vi "Read_Instr.vi"(8 "error in (no error)":errorcluster caption="entrée d'erreur (pas d'erreur)", 11 "Class Instrument Process en entrée":refnum<class "Class Instrument Process.lvclass">) -> (0 "error out":errorcluster caption="sortie d'erreur", 3 "Class Instrument Process en sortie":refnum<class "Class Instrument Process.lvclass">)   [LabVIEW 2020, in "Library Instrument & Equipement.lvlib" / "Library Instruments.lvlib" / "Class Instrument Process.lvclass"]
uses:
  Class Instrument Process.lvclass
  Class Instrument Process.lvclass/Class Instrument Process.ctl
  Instrument (Default)/Class Instrument (Default).lvclass
  Process/Process (Default)/Process (Default).lvclass
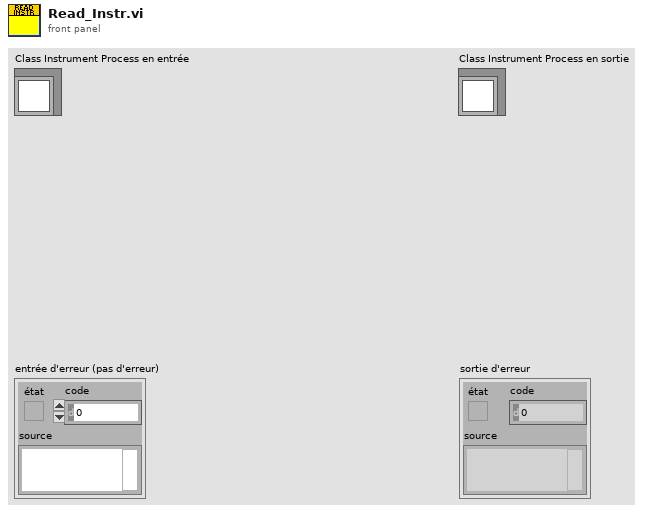
[diagram p1: front panel]
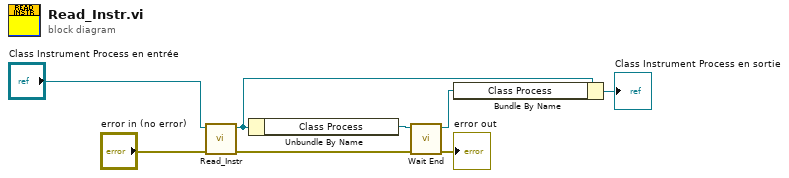
[diagram p0: block diagram]
diagram:
  n1 = call-parent "Read_Instr.vi"("error in (no error)"="error in (no error)", "Class Instrument (Default) en entrée"="Class Instrument Process en entrée") -> ("error out"=w1:errorcluster, "Class Instrument (Default) en sortie"=w3:refnum<class "Class Instrument Process.lvclass">)  [unwired: 8 in]
  n2 = Unbundle By Name(w3) -> ("Class Process"=w6:refnum<class "Process (Default).lvclass">)
  n3 = call-dynamic "Wait End.vi"("error in (no error)"=w1, "Process (Default) en entrée"=w6) -> ("error out"=→"error out":errorcluster, "Process (Default) en sortie"=w4:refnum<class "Process (Default).lvclass">)  [unwired: 8 in]
  n4 = Bundle By Name(cluster=w3, "Class Process"=w4) -> (→"Class Instrument Process en sortie":refnum<class "Class Instrument Process.lvclass">)
